vi "LED Spike.vi"(9 "ON/OFF":bool, 11 "State":enum16{"Open", "Run", "End"}(ring)=enum."Run") -> ()   [LabVIEW 2013]
uses:
  <vilib>/Rock Robotics/WPI/Relay/WPI_RelayDirection.ctl
  <vilib>/Rock Robotics/SystemInterfaces/DIO/FPGA_DIORelayChannel.ctl
  <vilib>/Rock Robotics/SystemInterfaces/Typedef/FPGA_TypedefDigitalModule.ctl
  <vilib>/Rock Robotics/WPI/Relay/WPI_RelayValue.ctl
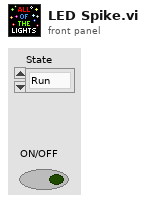
[diagram p1: front panel]
types:
  T1 = typedef "FPGA_TypedefDigitalModule.ctl" = enum16{"Digital Module 1", "Digital Module 2"}
  T2 = typedef "FPGA_DIORelayChannel.ctl" = enum8{"Relay 1", "Relay 2", "Relay 3", "Relay 4", "Relay 5", "Relay 6", "Relay 7", "Relay 8", "Invalid"}
  T3 = typedef "WPI_RelayDirection.ctl" = enum16{"Both directions", "Forward only", "Reverse only"}
  T4 = typedef "WPI_RelayValue.ctl" = enum16{"Off", "On", "Forward", "Reverse"}
  T5 = typedef "WPI_RelayDevRef.ctl" = cluster{"DevStatus":errorcluster, "Relay Channel":T2, "Digital Module":T1, "Relay Direction":T3}
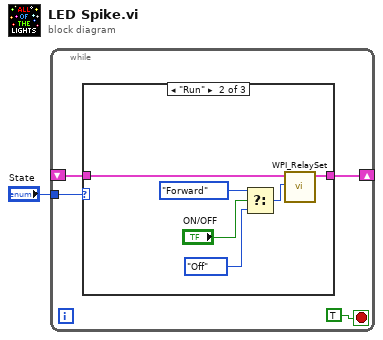
[diagram p0: block diagram]
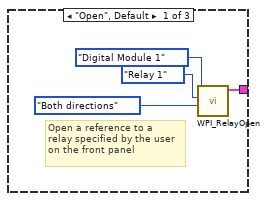
[diagram p2: hidden frame]
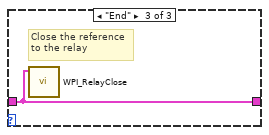
[diagram p3: hidden frame]
diagram:
  n1 = while {
    tunnel: "State" -> [w4]
    shift-right: [w3] -> _
    shift-left: _ -> [w2]
    stop <- TRUE stop-if-true
    n2 = case shown="\"Run\"" w4 {
      tunnel: [w7 w14 w16] -> w3
      tunnel: w2 -> [_ w15 w16]
      frame "Open", Default {
        # "Open a reference to a \nrelay specified by the user\non the front panel"
        n3 = call <vilib>:"WPI_RelayOpen.vi"("Relay Direction"=WPI_RelayDirection."Both directions" ("RelayDirection"), "Relay Channel"=FPGA_DIORelayChannel."Relay 1" ("RelayChannel"), "Digital Module (Module 1)"=FPGA_TypedefDigitalModule."Digital Module 1") -> ("RelayDevRef"=w7:T5)  [unwired: 1 in, 7 out]
      }
      frame "Run" {
        n4 = Select(t=WPI_RelayValue."Forward" ("RelayValue"), s="ON/OFF", f=WPI_RelayValue."Off" ("RelayValue")) -> (s? t:f=w11:T4)
        n5 = call <vilib>:"WPI_RelaySet.vi"("RelayValue"=w11, "RelayDevRef"=w15) -> ("RelayDevRef"=w14:T5)  [unwired: 1 in, 8 out]
      }
      frame "End" {
        # "Close the reference\nto the relay"
        n6 = call <vilib>:"WPI_RelayClose.vi"("RelayDevRef"=w16) -> ()  [unwired: 1 in, 10 out]
      }
    }
  }
